vi "uTTA_GetMaxMultiplier.vi"(8 "error in":errorcluster, 11 "VISA Refnum in":refnum<visa-resource-name>) -> (0 "error out":errorcluster, 3 "VISA Refnum out":refnum<visa-resource-name>, 5 "Max. Multiplier":i32, 7 "Received":string)   [LabVIEW 2021]
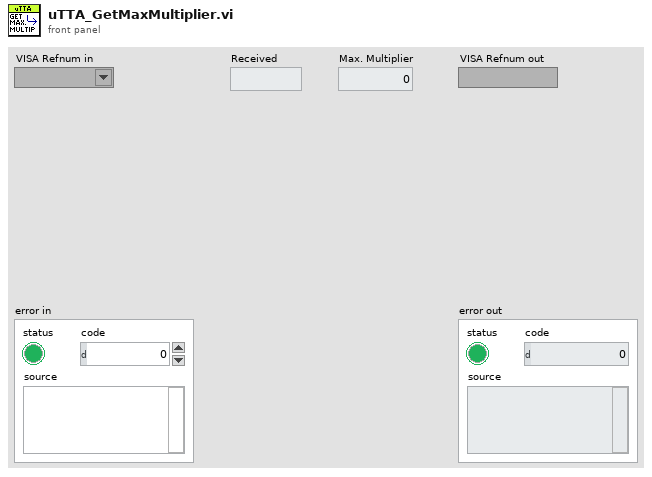
[diagram p1: front panel]
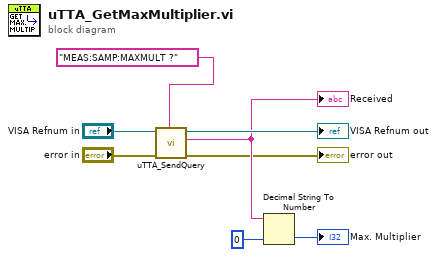
[diagram p0: block diagram]
diagram:
  n1 = call "uTTA_SendQuery.vi"("Send String"="MEAS:SAMP:MAXMULT ?" ("format string"), "error in (no error)"="error in", "VISA Refnum in"="VISA Refnum in") -> ("error out"=→"error out":errorcluster, "Received"=w2:string, "VISA Refnum out"=→"VISA Refnum out":refnum<visa-resource-name>)  [unwired: 6 in]
  "Received" <- w2
  n2 = Decimal String To Number(string=w2, default (0L)=0 ("default value 1")) -> (number=→"Max. Multiplier":i32)  [unwired: 1 in, 1 out]
